vi "CleanUpTemplateMethods.vi"() -> ()   [LabVIEW 2020]
uses:
  <vilib>/Utility/miscctls.llb/LVBoundsTypeDef.ctl
  <vilib>/Utility/miscctls.llb/LVPositionTypeDef.ctl
  <vilib>/Utility/traverseref.llb/TRef TravTarget.ctl
  <vilib>/Utility/miscctls.llb/LVPointTypeDef.ctl
  0c72b3e3-b306-43ed-a2af-d118a205124b.vi
  f0380e71-9b35-4e55-9a3a-ea54212ac198.vi
  <vilib>/ErrorRing/Error Ring.xnode
panel:
  in  "VI Name pattern":string[](array[string])=["methods"]
  in  "Folders to Search":path[](array[path])=[path "C:/Program Files (x86)/National Instruments/LabVIEW 2020/resource/Framework/Providers/Open_GDS/ClassProviders/Provider_LvNativeClass/Templates", path "C:/Program Files (x86)/National Instruments/LabVIEW 2020/resource/Framework/Providers/Open_GDS/ClassProviders/Provider_EndevoGOOP300/Templates", path "C:/Program Files (x86)/National Instruments/LabVIEW 2020/resource/Framework/Providers/Open_GDS/ClassProviders/Provider_EndevoGOOP400/Templates"]
  out "errors":errorcluster
  out "Property Out":dbl
  in  "Property In":dbl
  out "Object Out":refnum<class>
  in  "Object In":refnum<class>
  out "Error Out":errorcluster
  in  "Error In":errorcluster
  # "1) Set minimum size to this decoration\n2) Replace the Error in/out\n3) Place controls like this"
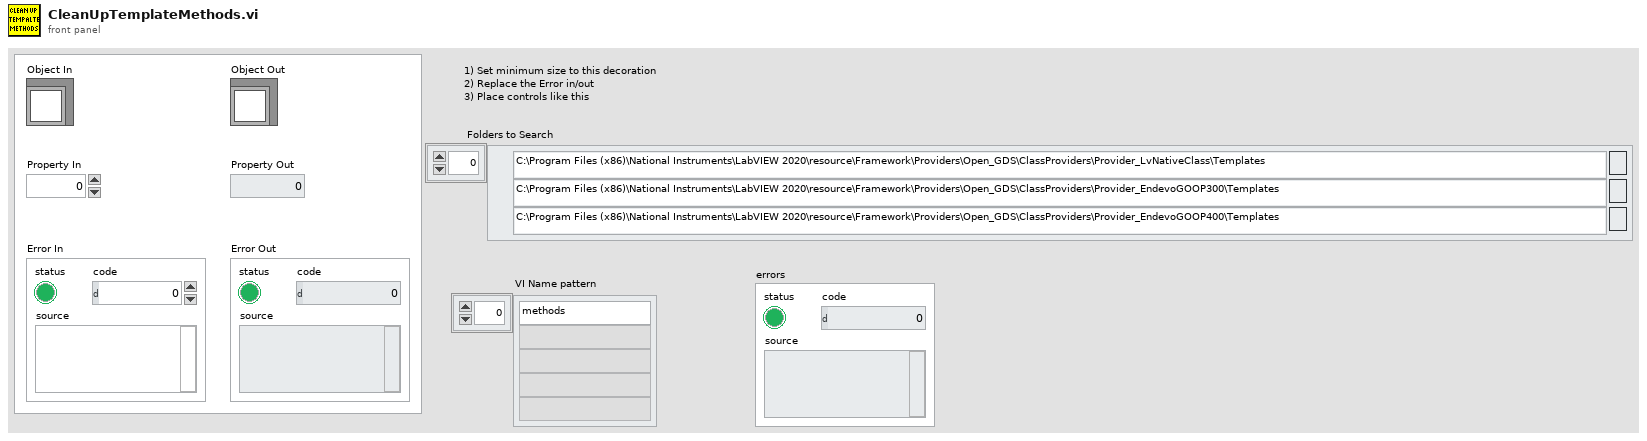
[diagram p1: front panel]
types:
  T1 = typedef "LVPositionTypeDef.ctl" = cluster{"Left":i32, "Top":i32}
  T2 = typedef "LVBoundsTypeDef.ctl" = cluster{"Width":u32, "Height":u32}
  T3 = cluster{"MinPanelSize":T2, "ObjectPositions":T1[], "FilesToModify":path[], "Index":u32, "TargetRef":refnum<vi>[], "SourceRef":refnum<vi>[], "SourceViRef":refnum<vi>, "ErrorIn/Out":path[], "TargetViRef":refnum<vi>, "Pane Color":u32}
  T4 = enum16{"Object In", "Object Out", "Property In", "Property Out", "Error In", "Error Out"}
  T5 = typedef "TRef TravTarget.ctl" = enum16{"FP", "BD", "Other"}
  T6 = enum32{"invalid VI type", "Standard VI", "Control VI", "Global VI", "Polymorphic VI", "Configuration VI", "SubSystem", "Facade VI", "Method VI", "Statechart Diagram VI"}
  T7 = typedef "LVPointTypeDef.ctl" = cluster{"Horizontal":i16, "Vertical":i16}
  T8 = enum16{"Object In", "Object Out", "Property In", "Property Out", "Error In", "Error Out"}[]
  T9 = cluster{"Left":i32, "Top":i32, "Width":u32, "Height":u32}
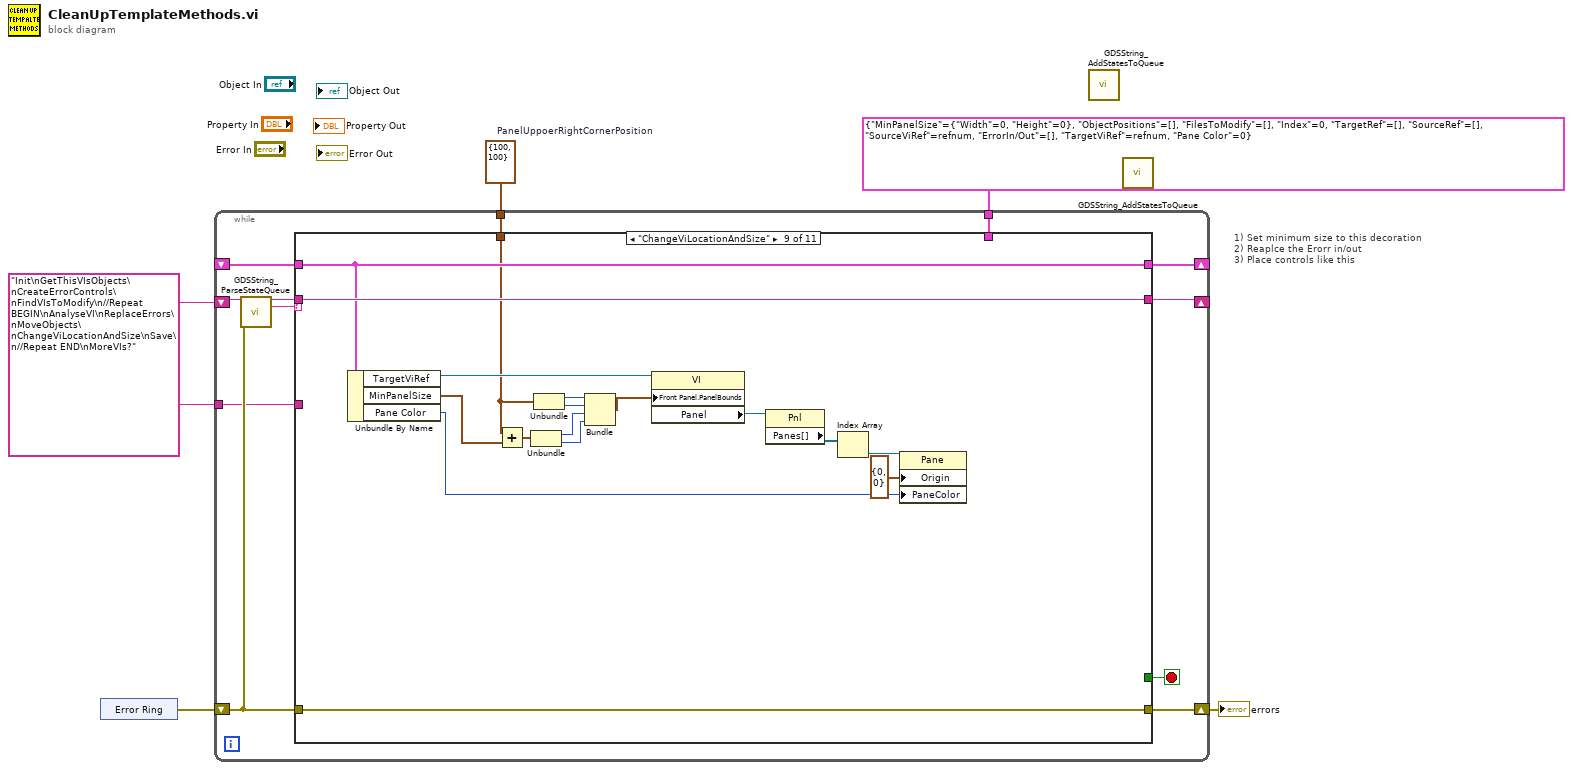
[diagram p0: block diagram]
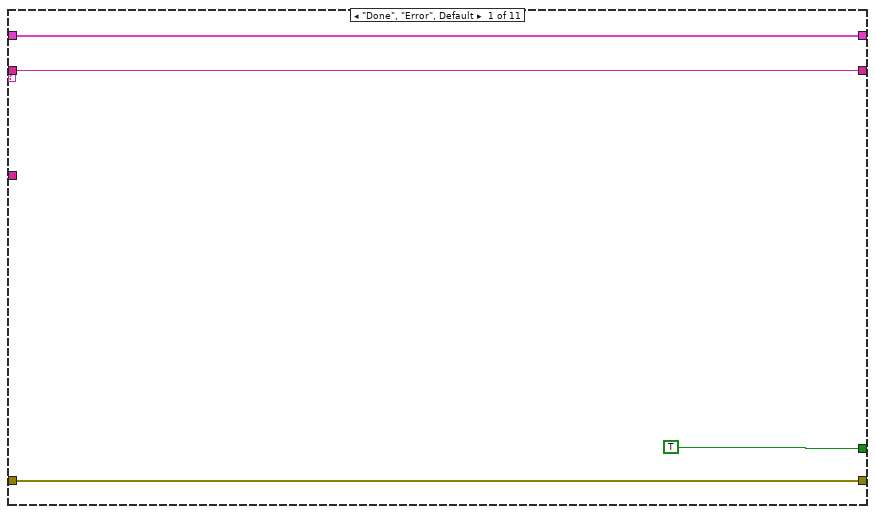
[diagram p2: hidden frame]
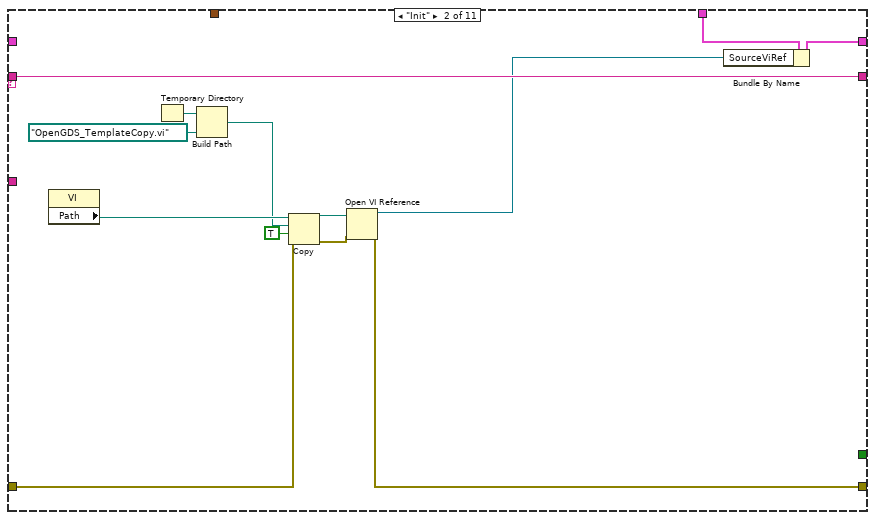
[diagram p3: hidden frame]
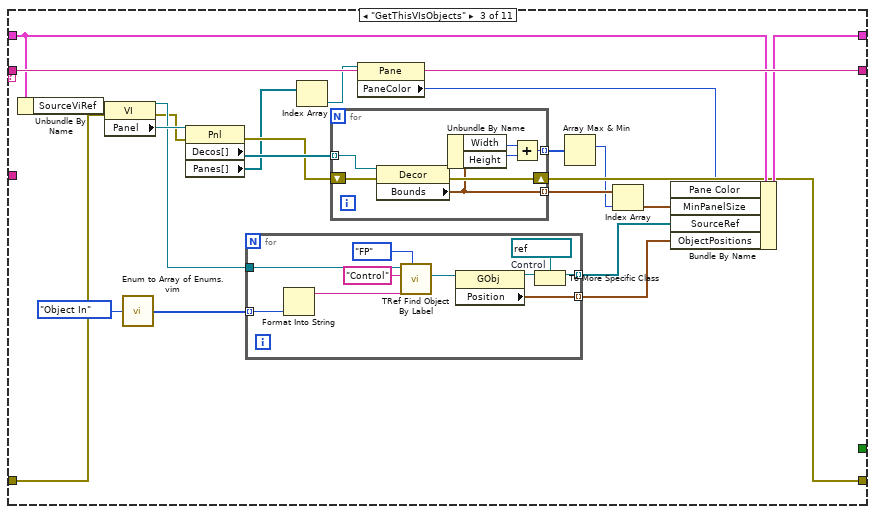
[diagram p4: hidden frame]
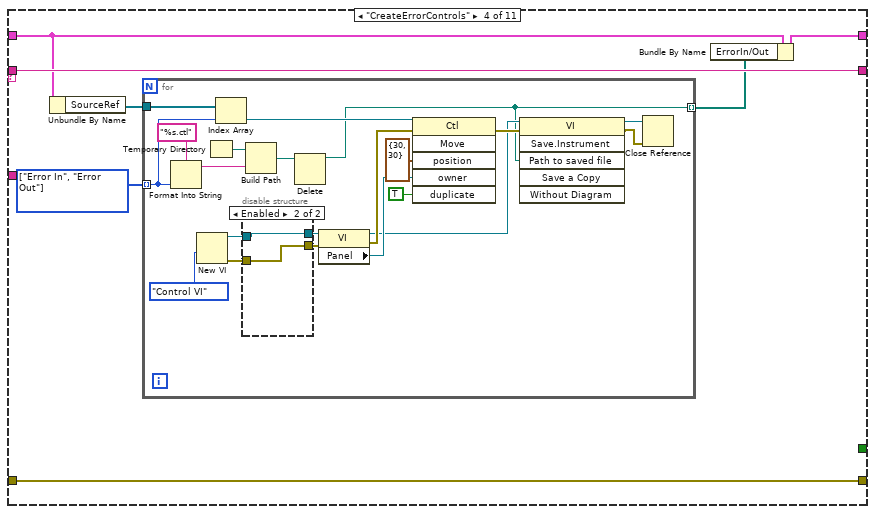
[diagram p5: hidden frame]
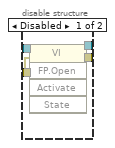
[diagram p6: hidden frame]
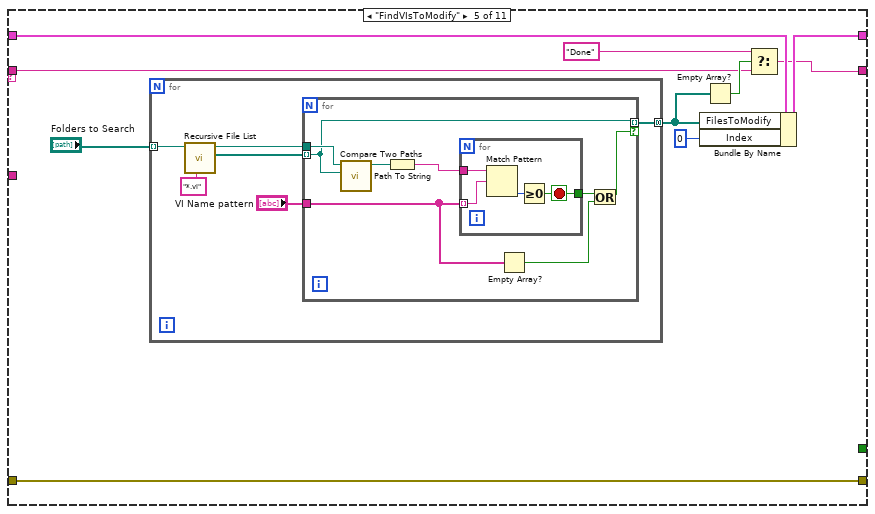
[diagram p7: hidden frame]
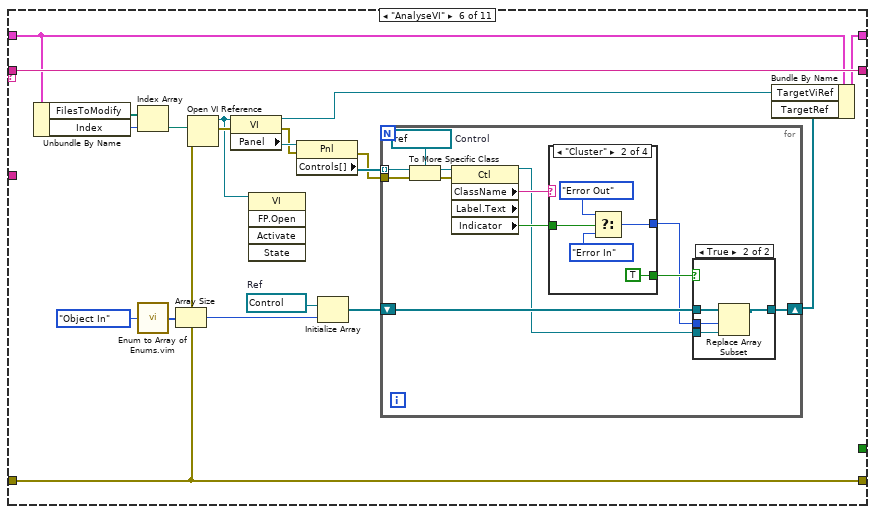
[diagram p8: hidden frame]
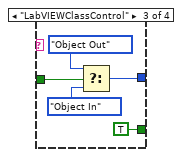
[diagram p11: hidden frame]
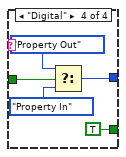
[diagram p12: hidden frame]
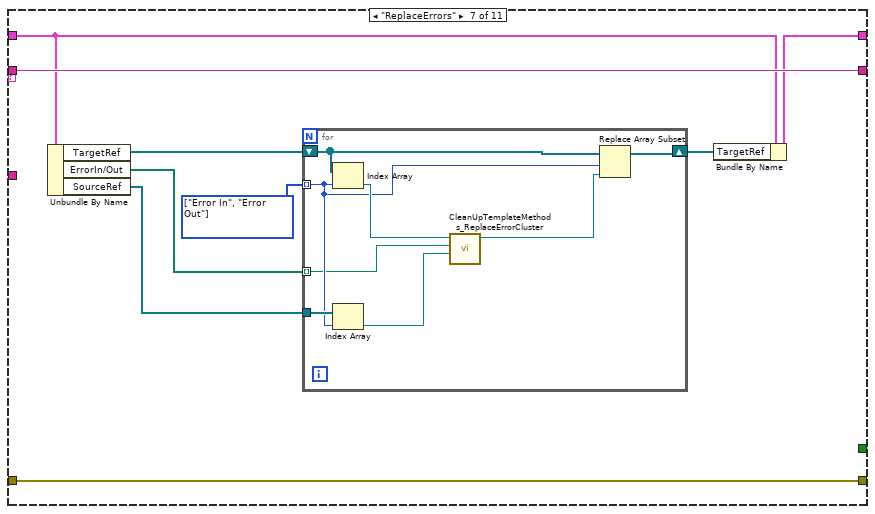
[diagram p13: hidden frame]
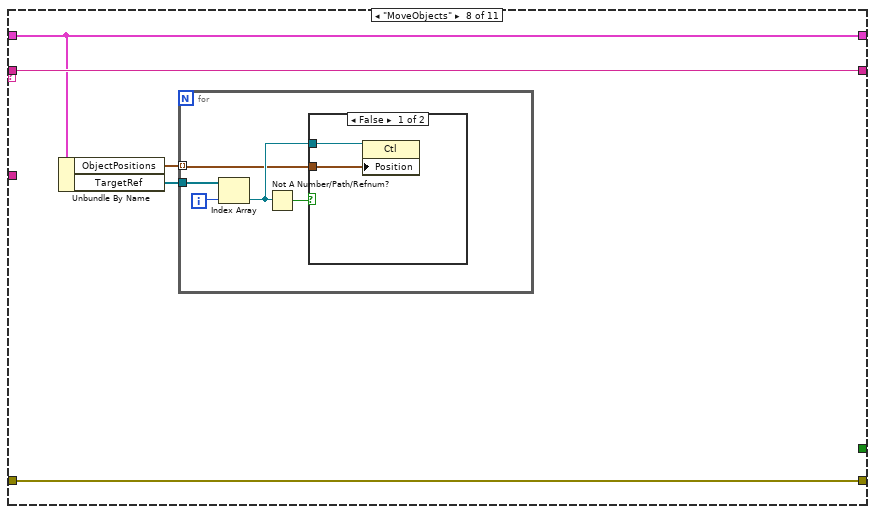
[diagram p14: hidden frame]
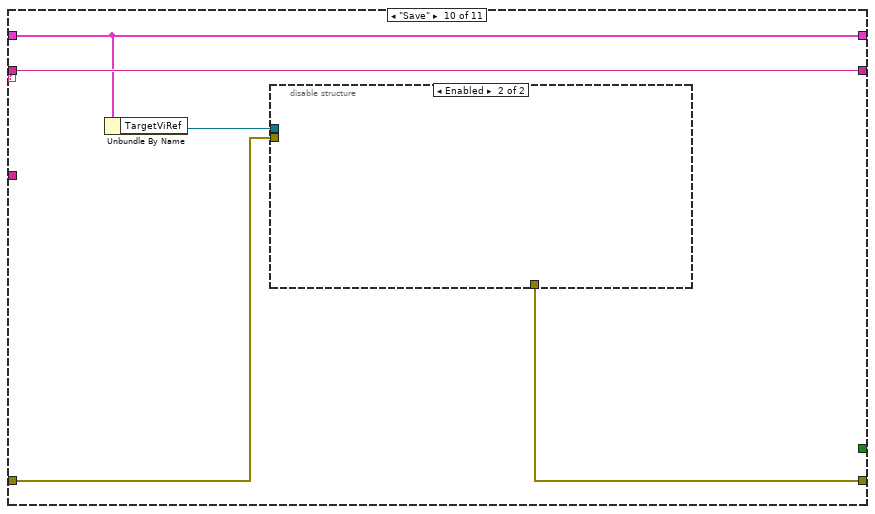
[diagram p16: hidden frame]
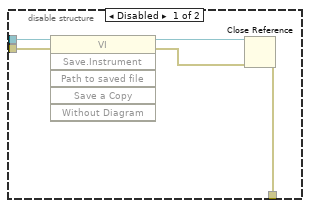
[diagram p17: hidden frame]
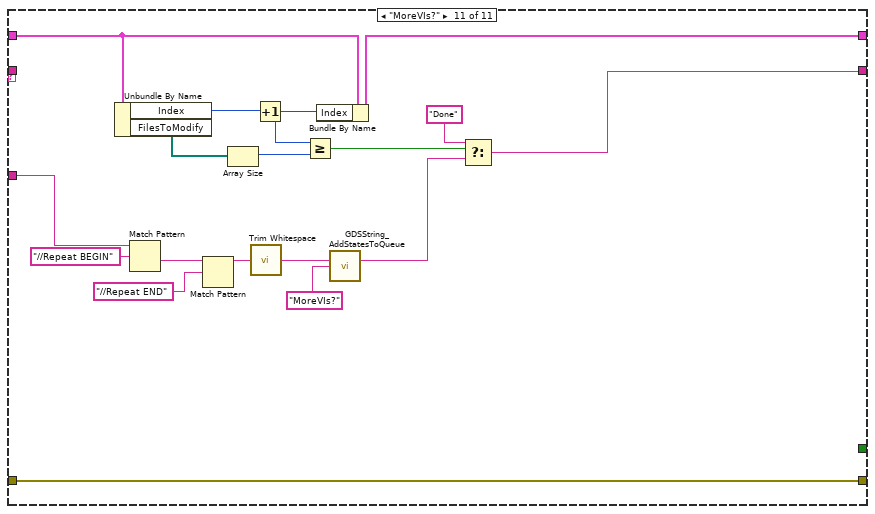
[diagram p18: hidden frame]
diagram:
  w2 = T1 {"Left"=100, "Top"=100}  # PanelUppoerRightCornerPosition
  w1 = "Init\nGetThisVIsObjects\nCreateErrorControls\nFindVIsToModify\n//Repeat BEGIN\nAnalyseVI\nReplaceErrors\nMoveObjects\nChangeViLocationAndSize\nSave\n//Repeat END\nMoreVIs?"
  # "1) Set minimum size to this decoration\n2) Reaplce the Erorr in/out\n3) Place controls like this"
  n1 = xnode "Error Ring"() -> ("error out"=w5:errorcluster)
  n2 = while {
    shift-right: [w11] -> _
    shift-left: w1 -> [w17]
    shift-right: [w14] -> w3
    shift-left: w5 -> [w15]
    shift-right: [w10] -> _
    shift-left: _ -> [w8]
    tunnel: T3 {"MinPanelSize"={"Width"=0, "Height"=0}, "ObjectPositions"=[], "FilesToModify"=[], "Index"=0, "TargetRef"=[], "SourceRef"=[], "SourceViRef"=refnum, "ErrorIn/Out"=[], "TargetViRef"=refnum, "Pane Color"=0} -> [w9]
    tunnel: w2 -> [w7]
    tunnel: w1 -> [w6]
    stop <- w13 stop-if-true
    n3 = call "GDSString_ParseStateQueue.vi"("State Queue"=w17, "Error In (no error)"=w15) -> ("Remaining States"=w12:string, "Current State"=w16:string)  [unwired: 9 in, 3 out]
    n4 = case shown="\"ChangeViLocationAndSize\"" w16 {
      tunnel: w15 -> [w21 w22 w42 w80 w117 w150 w196 w209 w233 w234 w261]
      tunnel: [w21 w23 w43 w80 w117 w150 w196 w209 w233 w235 w261] -> w14
      tunnel: [TRUE _ _ _ _ _ _ _ _ _ _] -> w13
      tunnel: [w19 w34 w56 w79 w109 w155 w195 w208 w232 w238 w247] -> w11
      tunnel: w12 -> [w19 w34 w56 w79 w110 w155 w195 w208 w232 w238 _]
      tunnel: [w18 w26 w53 w75 w114 w139 w190 w207 w231 w237 w258] -> w10
      tunnel: w9 -> [_ w33 _ _ _ _ _ _ _ _ _]
      tunnel: w8 -> [w18 _ w47 w77 w116 w154 w194 w207 w231 w237 w260]
      tunnel: w7 -> [_ _ _ _ _ _ _ _ w227 _ _]
      tunnel: w6 -> [_ _ _ _ _ _ _ _ _ _ w253]
      frame "Done", "Error", Default {
      }
      frame "Init" {
        n5 = property class="VI"() -> ("Path"=w31:path)  [unwired: 2 in, 2 out]
        n6 = Temporary Directory() -> (w32:path)
        n7 = Build Path(base path=w32, name or relative path=path "OpenGDS_TemplateCopy.vi") -> (appended path=w29:path)
        n8 = Copy(8:w22, 9:TRUE ("overwrite (F)"), 10:w29, 11:w31) -> (0:w24:errorcluster, 3:w27:path)  [unwired: 1 in, 1 out]
        n9 = Open VI Reference(vi path=w27, error in (no error)=w24) -> (vi reference=w25:refnum<vi>, error out=w23:errorcluster)  [unwired: 4 in]
        n10 = Bundle By Name(cluster=w33, "SourceViRef"=w25) -> (w26:T3)
      }
      frame "GetThisVIsObjects" {
        n11 = Unbundle By Name(w47) -> ("SourceViRef"=w46:refnum<vi>)
        n12 = property class="VI"(reference=w46, error in=w42) -> (reference out=w52:refnum<vi>, error out=w45:errorcluster, "Panel"=w55:refnum<vi>)
        n13 = call "Enum to Array of Enums.vim"("enum"=T4."Object In" ("Text Ring")) -> ("array of enums"=w49:T8)
        n14 = property class="Pnl"(reference=w55, error in=w45) -> (error out=w44:errorcluster, "Decos[]"=w54:refnum<vi>[], "Panes[]"=w37:refnum<vi>[])  [unwired: 1 out]
        n15 = for {
          tunnel: w52 -> [w73]
          tunnel: [w71] -> w51 mode=indexing
          tunnel: w49 -> [w68] mode=indexing
          tunnel: [w64] -> w48 mode=indexing
          w65 = refnum<vi> refnum  # Control
          n16 = Format Into String(w68) -> (resulting string=w67:string)  [unwired: 3 in, 1 out]
          n17 = call <vilib>:"TRef Find Object By Label.vi"("Label"=w67, "Traverse Target"=TRef_TravTarget."FP", "Class Name"="Control", "VI Ref"=w73) -> ("Found Obj Ref"=w72:refnum<vi>)  [unwired: 4 in, 3 out]
          n18 = property class="GObj"(reference=w72) -> (reference out=w66:refnum<vi>, "Position"=w71:T1)  [unwired: 1 in, 1 out]
          n19 = To More Specific Class(target class=w65, reference=w66) -> (specific class reference=w64:refnum<vi>)  [unwired: 1 in, 1 out]
        }
        n20 = Index Array(array=w37) -> (element=w36:refnum<vi>)  [unwired: 1 in]
        n21 = for {
          tunnel: w54 -> [w61] mode=indexing
          tunnel: [w60] -> w40 mode=indexing
          shift-right: [w62] -> w43
          shift-left: w44 -> [w63]
          tunnel: [w57] -> w41 mode=indexing
          n22 = property class="Decor"(reference=w61, error in=w63) -> (error out=w62:errorcluster, "Bounds"=w60:T2)  [unwired: 1 out]
          n23 = Unbundle By Name(w60) -> ("Width"=w59:u32, "Height"=w58:u32)
          n24 = Add(x=w59, y=w58) -> (x+y=w57:u32)
        }
        n25 = property class="Pane"(reference=w36) -> ("PaneColor"=w35:u32)  [unwired: 1 in, 2 out]
        n26 = Array Max & Min(array=w41) -> (max index (indices)=w39:i32)  [unwired: 3 out]
        n27 = Index Array(array=w40, index=w39) -> (element=w38:T2)
        n28 = Bundle By Name(cluster=w47, "Pane Color"=w35, "MinPanelSize"=w38, "SourceRef"=w48, "ObjectPositions"=w51) -> (w53:T3)
      }
      frame "CreateErrorControls" {
        w78 = T8 [enum."Error In", enum."Error Out"] items=["Object In", "Object Out", "Property In", "Property Out", "Error In", "Error Out"] ("Text Ring")
        n29 = Unbundle By Name(w77) -> ("SourceRef"=w76:refnum<vi>[])
        n30 = for {
          tunnel: w78 -> [w96] mode=indexing
          tunnel: w76 -> [w97]
          tunnel: [w81] -> w74 mode=indexing
          n31 = Format Into String(format string="%s.ctl", w96) -> (resulting string=w98:string)  [unwired: 2 in, 1 out]
          n32 = New VI(9:T6."Control VI" ("vi type (standard vi)")) -> (0:w85:errorcluster, 3:w86:refnum<vi>)  [unwired: 6 in]
          n33 = Temporary Directory() -> (w100:path)
          n34 = Index Array(array=w97, index=w96) -> (element=w95:refnum<vi>)
          n35 = disable-structure shown="Enabled" {
            disable-tunnel: w86 -> [w105 w107]
            disable-tunnel: w85 -> [w104 w106]
            disable-tunnel: [w103 w107] -> w84
            disable-tunnel: [w102 w106] -> w83
            frame Disabled {
              n36 = invoke class="VI" method="FP.Open"(reference=w105, error in=w104) -> (reference out=w103:refnum<vi>, error out=w102:errorcluster)  [unwired: 3 in, 3 out]
            }
            frame Enabled {
            }
          }
          n37 = Build Path(base path=w100, name or relative path=w98) -> (appended path=w82:path)
          n38 = Delete(path (use dialog)=w82) -> (deleted path=w81:path)  [unwired: 4 in, 2 out]
          n39 = property class="VI"(reference=w84, error in=w83) -> (reference out=w90:refnum<vi>, error out=w92:errorcluster, "Panel"=w94:refnum<vi>)
          n40 = invoke class="Ctl" method="Move"(reference=w95, error in=w92, "position"=T1 {"Left"=30, "Top"=30}, "owner"=w94, "duplicate"=TRUE ("Duplicate? (F)")) -> (error out=w91:errorcluster)  [unwired: 1 in, 5 out]
          n41 = invoke class="VI" method="Save.Instrument"(reference=w90, error in=w91, "Path to saved file"=w81) -> (reference out=w89:refnum<vi>, error out=w88:errorcluster)  [unwired: 3 in, 4 out]
          n42 = Close Reference(reference=w89, error in (no error)=w88) -> ()  [unwired: 1 out]
        }
        n43 = Bundle By Name(cluster=w77, "ErrorIn/Out"=w74) -> (w75:T3)
      }
      frame "FindVIsToModify" {
        n44 = for {
          tunnel: "Folders to Search" -> [w123] mode=indexing
          tunnel: [w119] -> w112 mode=concatenating
          n45 = call <vilib>:"Recursive File List.vi"("pattern"="*.vi", "Folder Path"=w123) -> ("All Files in Dir"=w121:path[], "dup Folder Path"=w118:path)  [unwired: 5 in, 3 out]
          n46 = for {
            tunnel: w121 -> [w126] mode=indexing
            tunnel: "VI Name pattern" -> [w131]
            tunnel: [w126] -> w119 mode=indexing if=w128
            tunnel: w118 -> [w127]
            n47 = call <vilib>:"Compare Two Paths.vi"("Path 2"=w126, "Path 1"=w127) -> ("Relative Path from 1 to 2"=w125:path)  [unwired: 6 in, 3 out]
            n48 = Path To String(path=w125) -> (string=w124:string)
            n49 = for {
              tunnel: w124 -> [w135]
              tunnel: w131 -> [w134] mode=indexing
              tunnel: [w132] -> w130
              stop <- w132 stop-if-true
              n50 = Match Pattern(string=w135, regular expression=w134) -> (offset past match=w133:i32)  [unwired: 1 in, 3 out]
              n51 = Greater Or Equal To 0?(x=w133) -> (x >= 0?=w132:bool)
            }
            n52 = Empty Array?(array=w131) -> (empty?=w129:bool)
            n53 = Or(x=w130, y=w129) -> (x .or. y?=w128:bool)
          }
        }
        n54 = Bundle By Name(cluster=w116, "FilesToModify"=w112, "Index"=u32 0) -> (w114:T3)
        n55 = Empty Array?(array=w112) -> (empty?=w111:bool)
        n56 = Select(t="Done", s=w111, f=w110) -> (s? t:f=w109:string)
      }
      frame "AnalyseVI" {
        w140 = refnum<vi> refnum  # Ref
        n57 = Unbundle By Name(w154) -> ("FilesToModify"=w153:path[], "Index"=w152:u32)
        n58 = Index Array(array=w153, index=w152) -> (element=w151:path)
        n59 = call "Enum to Array of Enums.vim"("enum"=T4."Object In" ("Text Ring")) -> ("array of enums"=w148:T8)
        n60 = Array Size(array=w148) -> (size(s)=w147:i32)
        n61 = Open VI Reference(vi path=w151, error in (no error)=w150) -> (vi reference=w136:refnum<vi>, error out=w144:errorcluster)  [unwired: 4 in]
        n62 = property class="VI"(reference=w136, error in=w144) -> (reference out=w137:refnum<vi>, error out=w142:errorcluster, "Panel"=w145:refnum<vi>)
        n63 = invoke class="VI" method="FP.Open"(reference=w136) -> ()  [unwired: 4 in, 5 out]
        n64 = property class="Pnl"(reference=w145, error in=w142) -> (error out=w141:errorcluster, "Controls[]"=w143:refnum<vi>[])  [unwired: 1 out]
        n65 = Initialize Array(w140, w147) -> (w146:refnum<vi>[])
        n66 = for {
          tunnel: w143 -> [w167] mode=indexing
          shift-right: [w160] -> w138
          shift-left: w146 -> [w161]
          tunnel: w141 -> [w158]
          w164 = refnum<vi> refnum  # Control
          n67 = To More Specific Class(target class=w164, reference=w167, error in=w158) -> (specific class reference=w165:refnum<vi>, error out=w157:errorcluster)
          n68 = property class="Ctl" props=["ClassName", "Label", "Text", "Indicator"](reference=w165, error in=w157) -> (reference out=w156:refnum<vi>, "ClassName"=w166:string, "Indicator"=w163:bool)  [unwired: 2 out]
          n69 = case shown="\"Cluster\"" w166 {
            tunnel: w163 -> [_ w177 w182 w187]
            tunnel: [_ w174 w179 w184] -> w159
            tunnel: [_ TRUE TRUE TRUE] -> w162
            frame Default {
            }
            frame "Cluster" {
              n70 = Select(t=T4."Error Out" ("Text Ring"), s=w177, f=T4."Error In" ("Text Ring")) -> (s? t:f=w174:T4)
            }
            frame "LabVIEWClassControl" {
              n71 = Select(t=T4."Object Out" ("Text Ring"), s=w182, f=T4."Object In" ("Text Ring")) -> (s? t:f=w179:T4)
            }
            frame "Digital" {
              n72 = Select(t=T4."Property Out" ("Text Ring"), s=w187, f=T4."Property In" ("Text Ring")) -> (s? t:f=w184:T4)
            }
          }
          n73 = case shown="True" w162 {
            tunnel: w161 -> [w168 w172]
            tunnel: [w168 w171] -> w160
            tunnel: w159 -> [_ w170]
            tunnel: w156 -> [_ w169]
            frame False {
            }
            frame True {
              n74 = Replace Array Subset(array=w172, new element=w169, index=w170) -> (w171:refnum<vi>[])
            }
          }
        }
        n75 = Bundle By Name(cluster=w154, "TargetViRef"=w137, "TargetRef"=w138) -> (w139:T3)
      }
      frame "ReplaceErrors" {
        w192 = T8 [enum."Error In", enum."Error Out"] items=["Object In", "Object Out", "Property In", "Property Out", "Error In", "Error Out"] ("Text Ring")
        n76 = Unbundle By Name(w194) -> ("TargetRef"=w193:refnum<vi>[], "ErrorIn/Out"=w191:path[], "SourceRef"=w188:refnum<vi>[])
        n77 = for {
          tunnel: w192 -> [w199] mode=indexing
          tunnel: w191 -> [w197] mode=indexing
          shift-right: [w202] -> w189
          shift-left: w193 -> [w203]
          tunnel: w188 -> [w200]
          n78 = Index Array(array=w203, index=w199) -> (element=w204:refnum<vi>)
          n79 = Index Array(array=w200, index=w199) -> (element=w198:refnum<vi>)
          n80 = call "CleanUpTemplateMethods_ReplaceErrorCluster.vi"("SourceErrorCluster"=w198, "NewErrorClusterCtlFile"=w197, "TargetErrorClusterToReplace"=w204) -> ("newErrorCluster"=w201:refnum<vi>)  [unwired: 8 in]
          n81 = Replace Array Subset(array=w203, new element=w201, index=w199) -> (w202:refnum<vi>[])
        }
        n82 = Bundle By Name(cluster=w194, "TargetRef"=w189) -> (w190:T3)
      }
      frame "MoveObjects" {
        n83 = Unbundle By Name(w207) -> ("ObjectPositions"=w206:T1[], "TargetRef"=w205:refnum<vi>[])
        n84 = for {
          tunnel: w206 -> [w210] mode=indexing
          tunnel: w205 -> [w214]
          i -> [w213]
          n85 = Index Array(array=w214, index=w213) -> (element=w211:refnum<vi>)
          n86 = Not A Number/Path/Refnum?(number/path/refnum=w211) -> (NaN/Path/Refnum?=w212:bool)
          n87 = case shown="False" w212 {
            tunnel: w211 -> [w216 _]
            tunnel: w210 -> [w215 _]
            frame False {
              n88 = property class="Ctl"(reference=w216, "Position"=w215) -> ()  [unwired: 1 in, 2 out]
            }
            frame True {
            }
          }
        }
      }
      frame "ChangeViLocationAndSize" {
        n89 = Unbundle By Name(w231) -> ("TargetViRef"=w230:refnum<vi>, "MinPanelSize"=w226:T2, "Pane Color"=w217:u32)
        n90 = Add(x=w227, y=w226) -> (x+y=w225:T2)
        n91 = Unbundle(w225) -> ("Width"=w224:u32, "Height"=w223:u32)
        n92 = Unbundle(w227) -> ("Left"=w229:i32, "Top"=w228:i32)
        n93 = Bundle("Left"=w229, "Top"=w228, "Width"=w224, "Height"=w223) -> (w222:T9)  [unwired: 1 in]
        n94 = property class="VI"(reference=w230, "Front Panel.PanelBounds"=w222) -> ("Panel"=w221:refnum<vi>)  [unwired: 1 in, 2 out]
        n95 = property class="Pnl"(reference=w221) -> ("Panes[]"=w220:refnum<vi>[])  [unwired: 1 in, 2 out]
        n96 = Index Array(array=w220) -> (element=w219:refnum<vi>)  [unwired: 1 in]
        n97 = property class="Pane"(reference=w219, "Origin"=T7 {"Horizontal"=0, "Vertical"=0}, "PaneColor"=w217) -> ()  [unwired: 1 in, 2 out]
      }
      frame "Save" {
        n98 = Unbundle By Name(w237) -> ("TargetViRef"=w236:refnum<vi>)
        n99 = disable-structure shown="Enabled" {
          disable-tunnel: w236 -> [w243 _]
          disable-tunnel: [w240 _] -> w235
          disable-tunnel: w234 -> [w239 _]
          frame Disabled {
            n100 = invoke class="VI" method="Save.Instrument"(reference=w243, error in=w239) -> (reference out=w242:refnum<vi>, error out=w241:errorcluster)  [unwired: 4 in, 4 out]
            n101 = Close Reference(reference=w242, error in (no error)=w241) -> (error out=w240:errorcluster)
          }
          frame Enabled {
          }
        }
      }
      frame "MoreVIs?" {
        n102 = Unbundle By Name(w260) -> ("Index"=w259:u32, "FilesToModify"=w257:path[])
        n103 = Match Pattern(string=w253, regular expression="//Repeat BEGIN") -> (after substring=w251:string)  [unwired: 1 in, 3 out]
        n104 = Match Pattern(string=w251, regular expression="//Repeat END") -> (before substring=w249:string)  [unwired: 1 in, 3 out]
        n105 = Array Size(array=w257) -> (size(s)=w255:i32)
        n106 = call <vilib>:"Trim Whitespace.vi"("string"=w249) -> ("trimmed string"=w246:string)  [unwired: 1 in]
        n107 = Increment(x=w259) -> (x+1=w256:u32)
        n108 = Greater Or Equal?(x=w256, y=w255) -> (x >= y?=w254:bool)
        n109 = Bundle By Name(cluster=w260, "Index"=w256) -> (w258:T3)
        n110 = call "GDSString_AddStatesToQueue.vi"("State(s) in (\"\")"=w246, "State(s) at Back (\"\")"="MoreVIs?") -> ("States Out"=w245:string)  [unwired: 13 in]
        n111 = Select(t="Done", s=w254, f=w245) -> (s? t:f=w247:string)
      }
    }
  }
  "errors" <- w3
  n112 = call "GDSString_AddStatesToQueue.vi"() -> ()  [unwired: 15 in, 1 out]
  n113 = call "GDSString_AddStatesToQueue.vi"() -> ()  [unwired: 15 in, 1 out]
